vi "Get HTTP Servo Info.vi"(8 "error in (no error)":errorcluster, 11 "Node in":refnum<class "Node Config.lvclass">) -> (0 "error out":errorcluster, 2 "HTTP Server Info":T1, 3 "Node out":refnum<class "Node Config.lvclass">)   [LabVIEW 2020, in "VectoConfig.lvlib" / "Node Config.lvclass"]
uses:
  Node Config.lvclass
  Node Config.lvclass/Node Config.ctl
  HTTP Server Info.ctl
  VectoConfig/VectoConfig.lvlib
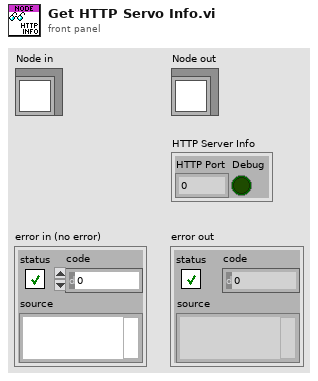
[diagram p1: front panel]
types:
  T1 = typedef "VectoConfig.lvlib/HTTP Server Info.ctl" = cluster{"HTTP Port":u16, "Debug":bool}
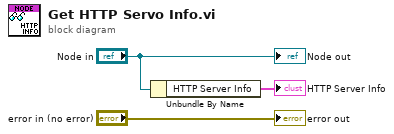
[diagram p0: block diagram]
diagram:
  n1 = Unbundle By Name("Node in") -> ("HTTP Server Info"=→"HTTP Server Info":T1)
  "error out" <- "error in (no error)"
  "Node out" <- "Node in"
